vi "ThreadCfg - Control Dialog UI.vi"(7 "rxPacket?":bool, 9 "threadManagement":T2, 10 "threadPeriodRef":T3=enum."Async") -> (0 "priorityState":T1(ring), 1 "pclDecimationState":T1(ring), 2 "loopPeriodState":T1(ring), 4 "processorState":T1(ring))   [LabVIEW 2019, in "UDP-Custom-Device System Explorer.lvlib"]
uses:
  UDP-Custom-Device System Explorer.lvlib
  Types/Threading/Thread Sync Reference.ctl
  Shared/Types/Shared - Thread Management.ctl
  Shared/UDP-Custom-Device Shared.lvlib
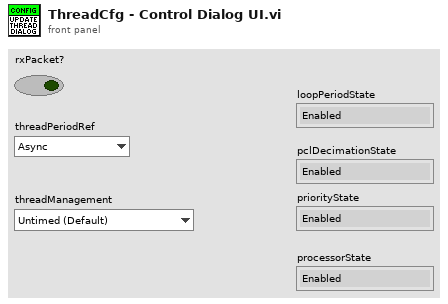
[diagram p1: front panel]
types:
  T1 = enum8{"Enabled", "Disabled", "Disabled and Grayed Out"}
  T2 = typedef "UDP-Custom-Device Shared.lvlib/Shared - Thread Management.ctl" = enum16{"Untimed (Default)", "Timed (High Priority)"}
  T3 = typedef "UDP-Custom-Device System Explorer.lvlib/Thread Sync Reference.ctl" = enum16{"PCL", "Async"}
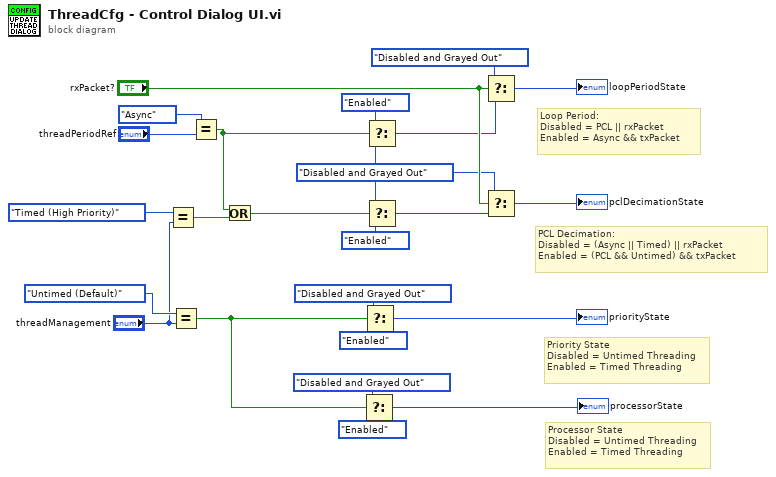
[diagram p0: block diagram]
diagram:
  w14 = T1."Disabled and Grayed Out" ("Disabled")
  # "Processor State\nDisabled = Untimed Threading\nEnabled = Timed Threading"
  # "Loop Period:\nDisabled = PCL || rxPacket\nEnabled = Async && txPacket"
  # "PCL Decimation:\nDisabled = (Async || Timed) || rxPacket\nEnabled = (PCL && Untimed) && txPacket"
  # "Priority State\nDisabled = Untimed Threading\nEnabled = Timed Threading"
  n1 = Equal?(x=Shared_-_Thread_Management."Timed (High Priority)", y="threadManagement") -> (x = y?=w6:bool)
  n2 = Equal?(x=Shared_-_Thread_Management."Untimed (Default)", y="threadManagement") -> (x = y?=w1:bool)
  n3 = Equal?(x=Thread_Sync_Reference."Async", y="threadPeriodRef") -> (x = y?=w5:bool)
  n4 = Or(x=w5, y=w6) -> (x .or. y?=w13:bool)
  n5 = Select(t=T1."Disabled and Grayed Out" ("Disabled"), s=w1, f=T1."Enabled" ("Disabled")) -> (s? t:f=→"processorState":T1)
  n6 = Select(t=T1."Disabled and Grayed Out" ("Disabled"), s=w1, f=T1."Enabled" ("Disabled")) -> (s? t:f=→"priorityState":T1)
  n7 = Select(t=T1."Enabled" ("Disabled"), s=w5, f=w14) -> (s? t:f=w15:T1)
  n8 = Select(t=w14, s=w13, f=T1."Enabled" ("Disabled")) -> (s? t:f=w16:T1)
  n9 = Select(t=T1."Disabled and Grayed Out" ("Disabled"), s="rxPacket?", f=w15) -> (s? t:f=→"loopPeriodState":T1)
  n10 = Select(t=w14, s="rxPacket?", f=w16) -> (s? t:f=→"pclDecimationState":T1)
